vi "CreateEventFile.vi"(8 "error in (no error)":errorcluster, 11 "object in":refnum<class "EventLogger_Actor.lvclass">) -> (0 "error out":errorcluster, 3 "object out":refnum<class "EventLogger_Actor.lvclass">)   [LabVIEW 2014, in "EventLogger_Actor.lvlib" / "EventLogger_Actor.lvclass"]
uses:
  EventLogger_Actor.lvclass
  EventLogger_Actor.lvclass/EventLogger_Actor.ctl
panel:
  # "BSD 2-Clause License\n\nCopyright (c) 2018, Ajay www.digiajay.com\nAll rights reserved.\n\nRedistribution and use in source and binary forms, with or without\nmodification, are permitted provided that the following conditions are met:\n\n* Redistributions of source code must retain the above copyright notice, this\n  list of conditions and the following disclaimer.\n\n* Redistributions in binary form must reproduce the above copyright notice,\n  this list of conditions and the following disclaimer in the documentation\n  and/or other materials provided with the distribution.\n\nTHIS SOFTWARE IS PROVIDED BY THE COPYRIGHT HOLDERS AND CONTRIBUTORS \"AS IS\"\nAND ANY EXPRESS OR IMPLIED WARRANTIES, INCLUDING, BUT NOT LIMITED TO, THE\nIMPLIED WARRANTIES OF MERCHANTABILITY AND FITNESS FOR A PARTICULAR PURPOSE ARE\nDISCLAIMED. IN NO EVENT SHALL THE COPYRIGHT HOLDER OR CONTRIBUTORS BE LIABLE\nFOR ANY DIRECT, INDIRECT, INCIDENTAL, SPECIAL, EXEMPLARY, OR CONSEQUENTIAL\nDAMAGES (INCLUDING, BUT NOT LIMITED TO, PROCUREMENT OF SUBSTITUTE GOODS OR\nSERVICES; LOSS OF USE, DATA, OR PROFITS; OR BUSINESS INTERRUPTION) HOWEVER\nCAUSED AND ON ANY THEORY OF LIABILITY, WHETHER IN CONTRACT, STRICT LIABILITY,\nOR TORT (INCLUDING NEGLIGENCE OR OTHERWISE) ARISING IN ANY WAY OUT OF THE USE\nOF THIS SOFTWARE, EVEN IF ADVISED OF THE POSSIBILITY OF SUCH DAMAGE."
  # "Connector Pane"
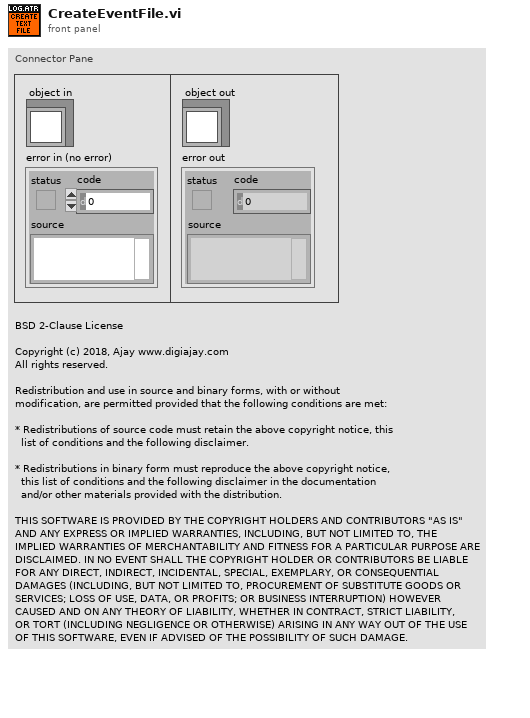
[diagram p1: front panel]
types:
  T1 = enum16{"open", "replace", "create", "open or create", "replace or create", "replace or create with confirmation"}
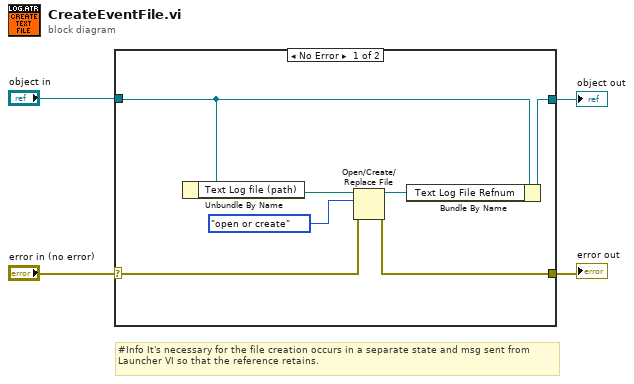
[diagram p0: block diagram]
diagram:
  # "#Info It's necessary for the file creation occurs in a separate state and msg sent from Launcher VI so that the reference retains."
  n1 = case shown="No Error" "error in (no error)" {
    selector: "error in (no error)" -> [w9 w13]
    tunnel: [w8 w13] -> w3
    tunnel: [w10 w12] -> w1
    tunnel: "object in" -> [w11 w12]
    frame No Error {
      n2 = Unbundle By Name(w11) -> ("Text Log file (path)"=w7:path)
      n3 = Open/Create/Replace File(file path (use dialog)=w7, error in=w9, operation (0:open)=T1."open or create") -> (refnum out=w6:refnum<file>, error out=w8:errorcluster)  [unwired: 3 in, 1 out]
      n4 = Bundle By Name(cluster=w11, "Text Log File Refnum"=w6) -> (w10:refnum<class "EventLogger_Actor.lvclass">)
    }
    frame Error {
    }
  }
  "error out" <- w3
  "object out" <- w1
